vi "Dawson's Integral.vi"(3 "x":dbl format="%.2f") -> (1 "daw(x)":dbl format="%.2f")   [LabVIEW 2020, in "NI_Gmath.lvlib"]
doc: "Computes the Dawson integral."
uses:
  <vilib>/gmath/NI_Gmath.lvlib
  <resource>/lvanlys.dll
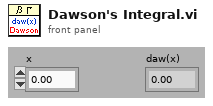
[diagram p1: front panel]
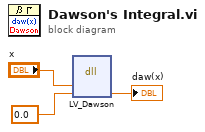
[diagram p0: block diagram]
diagram:
  n1 = dll-call lib="e:/builds/penguin/labview/branches/2020/dev/dist/resource/lvanlys.*" fn="LV_Dawson"("x"="x", "dawson(x)"=0.0 ("Erf")) -> ("dawson(x)"=→"daw(x)":dbl)  [unwired: 5 in, 2 out]
